vi "Idle Trans.vi"(8 "error in (no error)":errorcluster caption="错误输入（无错误）", 11 "SM Data In":T1) -> (0 "error out":errorcluster caption="错误输出", 1 "Trans Next?":bool, 3 "SM Data Out":T1)   [LabVIEW 2013, in "标准状态机模板.lvlib"]
uses:
  Control/SM Data.ctl
  Control/State.ctl
  Control/Input Data.ctl
  Control/Output Data.ctl
  Control/Internal Data.ctl
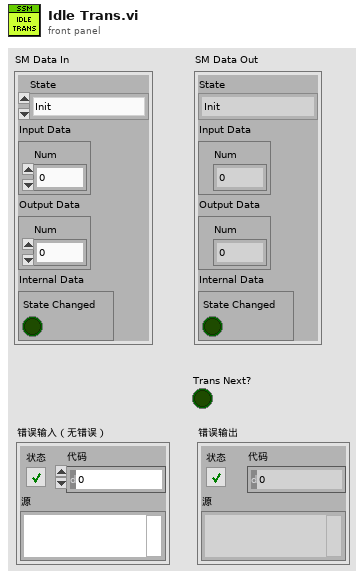
[diagram p1: front panel]
types:
  T1 = typedef "标准状态机模板.lvlib/SM Data.ctl" = cluster{"State":T2, "Input Data":T3, "Output Data":T4, "Internal Data":T5}
  T2 = typedef "标准状态机模板.lvlib/State.ctl" = enum16{"Init", "Idle"}
  T3 = typedef "标准状态机模板.lvlib/Input Data.ctl" = cluster{"Num":dbl}
  T4 = typedef "标准状态机模板.lvlib/Output Data.ctl" = cluster{"Num":dbl}
  T5 = typedef "标准状态机模板.lvlib/Internal Data.ctl" = cluster{"State Changed":bool}
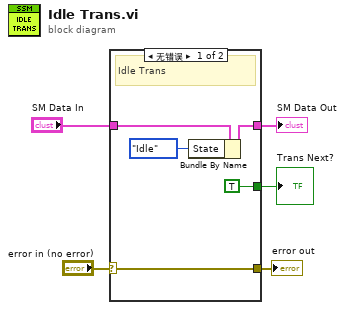
[diagram p0: block diagram]
diagram:
  n1 = case shown="无错误" "error in (no error)" {
    selector: "error in (no error)" -> [w10 w12]
    tunnel: [w10 w12] -> w4
    tunnel: "SM Data In" -> [w9 w11]
    tunnel: [w7 w11] -> w2
    tunnel: [TRUE _] -> w1
    frame No Error {
      # "Idle Trans"
      n2 = Bundle By Name(cluster=w9, "State"=State."Idle") -> (w7:T1)
    }
    frame Error {
    }
  }
  "SM Data Out" <- w2
  "error out" <- w4
  "Trans Next?" <- w1
